vi "Reopen Panel.vi"(8 "error in (no error)":errorcluster, 11 "Console in":refnum<class "Console.lvclass">) -> (0 "error out":errorcluster, 3 "Console out":refnum<class "Console.lvclass">)   [LabVIEW 2015, in "EditPanel API.lvlib" / "Console.lvclass"]
uses:
  Console.lvclass
  Console.lvclass/Console.ctl
  Console Reply/Console Reply/Console Reply.lvclass/Console Reply.ctl
  Console Reply/Console Reply/Console Reply.lvclass
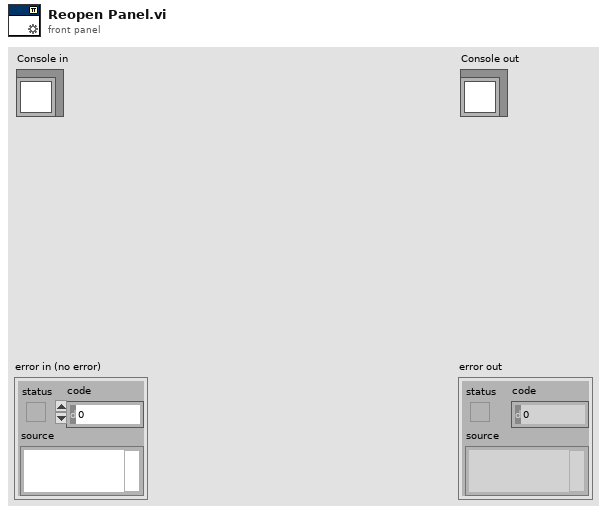
[diagram p1: front panel]
types:
  T1 = enum32{"Bad", "Idle", "Run top level", "Running"}
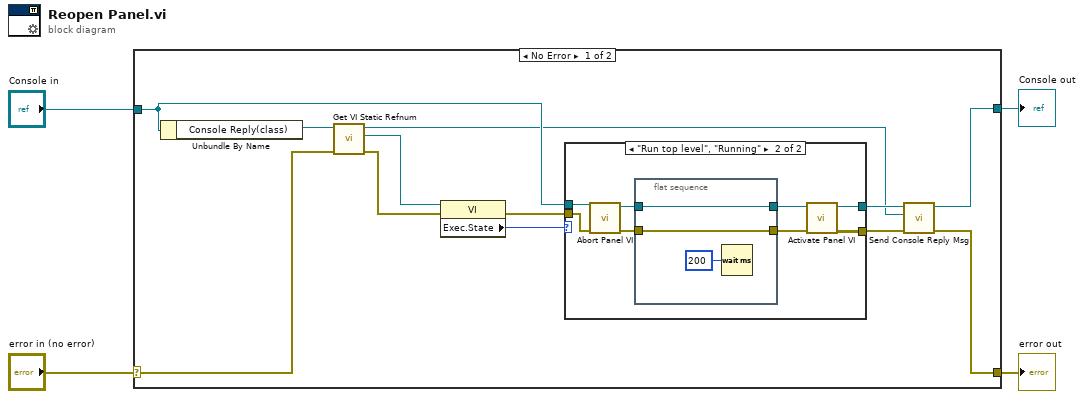
[diagram p0: block diagram]
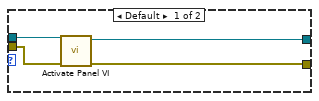
[diagram p2: hidden frame]
diagram:
  n1 = case shown="No Error" "error in (no error)" {
    selector: "error in (no error)" -> [w10 w33]
    tunnel: [w13 w33] -> w3
    tunnel: [w14 w32] -> w1
    tunnel: "Console in" -> [w12 w32]
    frame No Error {
      n2 = Unbundle By Name(w12) -> ("Console Reply(class)"=w11:refnum<class "Console Reply.lvclass">)
      n3 = call "Get VI Static Refnum.vi"("error in (no error)"=w10, "Console Reply in"=w11) -> ("error out"=w9:errorcluster, "VI Static Refnum"=w6:refnum<vi>, "Console Reply out"=w5:refnum<class "Console Reply.lvclass">)  [unwired: 7 in]
      n4 = property class="VI"(reference=w6, error in=w9) -> (error out=w15:errorcluster, "Exec.State"=w16:T1)  [unwired: 1 out]
      n5 = case shown="\"Run top level\", \"Running\"" w16 {
        tunnel: w15 -> [w20 w28]
        tunnel: [w19 w26] -> w7
        tunnel: [w18 w27] -> w8
        tunnel: w12 -> [w17 w25]
        frame Default {
          n6 = call "Activate Panel VI.vi"("error in (no error)"=w20, "Console in"=w17) -> ("error out"=w19:errorcluster, "Console out"=w18:refnum<class "Console.lvclass">)  [unwired: 8 in]
        }
        frame "Run top level", "Running" {
          n7 = call "Abort Panel VI.vi"("error in (no error)"=w28, "Console in"=w25) -> ("error out"=w23:errorcluster, "Console out"=w24:refnum<class "Console.lvclass">)  [unwired: 8 in]
          n8 = flat-sequence {
            tunnel: w24 -> [w30]
            tunnel: w23 -> [w31]
            tunnel: [w31] -> w22
            tunnel: [w30] -> w21
            frame #0 {
              n9 = Wait (ms)(milliseconds to wait=u32 200) -> ()  [unwired: 1 out]
            }
          }
          n10 = call "Activate Panel VI.vi"("error in (no error)"=w22, "Console in"=w21) -> ("error out"=w26:errorcluster, "Console out"=w27:refnum<class "Console.lvclass">)  [unwired: 8 in]
        }
      }
      n11 = call "Send Console Reply Msg.vi"("error in (no error)"=w7, "Console Reply"=w5, "Console in"=w8) -> ("error out"=w13:errorcluster, "Console out"=w14:refnum<class "Console.lvclass">)  [unwired: 7 in]
    }
    frame Error {
    }
  }
  "error out" <- w3
  "Console out" <- w1
